vi "file list from temperatures file.vi"(11 "file path":path=path "/snowfall/Users/arcadi/Desktop/Ultrasound/Experiment/YBCO_4/Round1/Sweep12/June_2011/062511/221.16400K_300_3100_001_062511.dat") -> (0 "timestamp":dbl[](array[numeric]), 2 "sweep file name array":T1[](array[typedef]), 3 "temperatures":dbl[](array[numeric]))   [LabVIEW 2010]
uses:
  sweep file name.ctl
  <vilib>/regexp/Match Regular Expression.xnode
  <vilib>/Utility/file.llb/Read From Spreadsheet File (string).vi
panel:
  in  "dummy 2":T1={"temperature"=0.0, "temperature str"="", "file path"=path "/snowfall/Users/arcadi/Desktop/Ultrasound/Experiment/YBCO_4/Round1/Sweep12/June_2011/062511/221.16400K_300_3100_001_062511.dat", "last mod"=timestamp(0 s since 1904-01-01), "file name str"="", "mod time(min)"=0.0}
  in  "dummy":T1={"temperature"=0.0, "temperature str"="", "file path"=path "/snowfall/Users/arcadi/Desktop/Ultrasound/Experiment/YBCO_4/Round1/Sweep12/June_2011/062511/221.16400K_300_3100_001_062511.dat", "last mod"=timestamp(0 s since 1904-01-01), "file name str"="", "mod time(min)"=0.0}
  in  "sweep file name":T1={"temperature"=0.0, "temperature str"="", "file path"=path "/snowfall/Users/arcadi/Desktop/Ultrasound/Experiment/YBCO_4/Round1/Sweep12/June_2011/062511/221.16400K_300_3100_001_062511.dat", "last mod"=timestamp(0 s since 1904-01-01), "file name str"="", "mod time(min)"=0.0}
  in  "file path OK":bool=TRUE
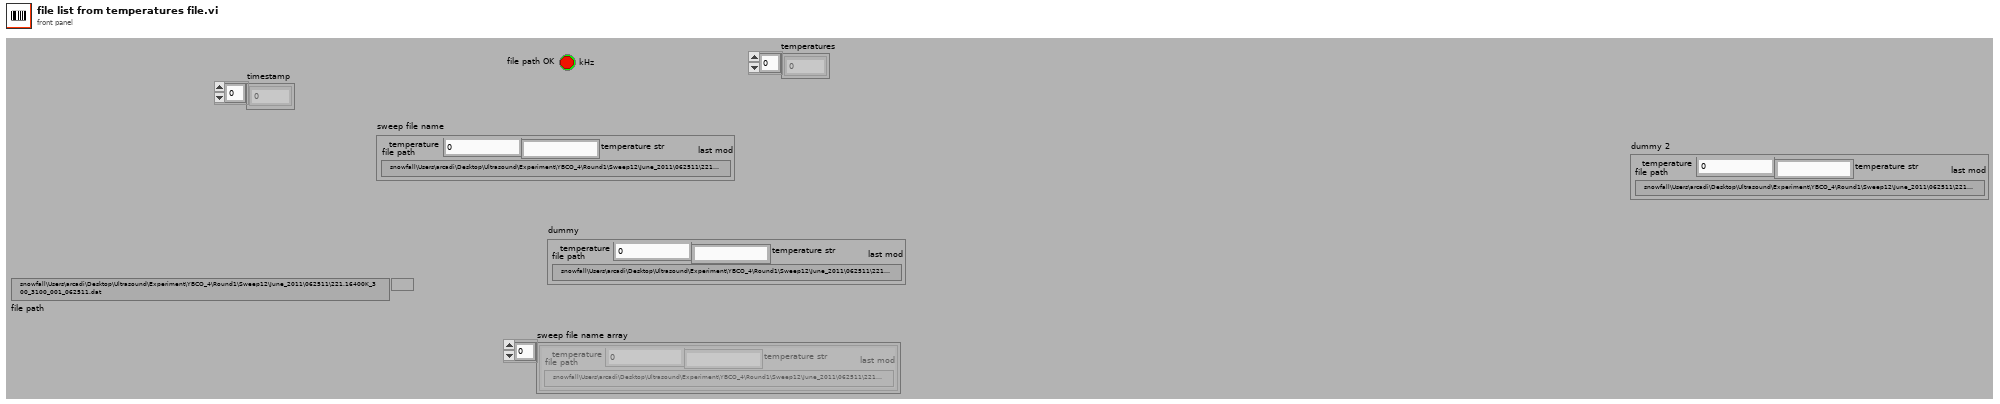
[diagram p1: front panel]
types:
  T1 = typedef "sweep file name.ctl" = cluster{"temperature":dbl, "temperature str":string, "file path":path, "last mod":timestamp, "file name str":string, "mod time(min)":dbl}
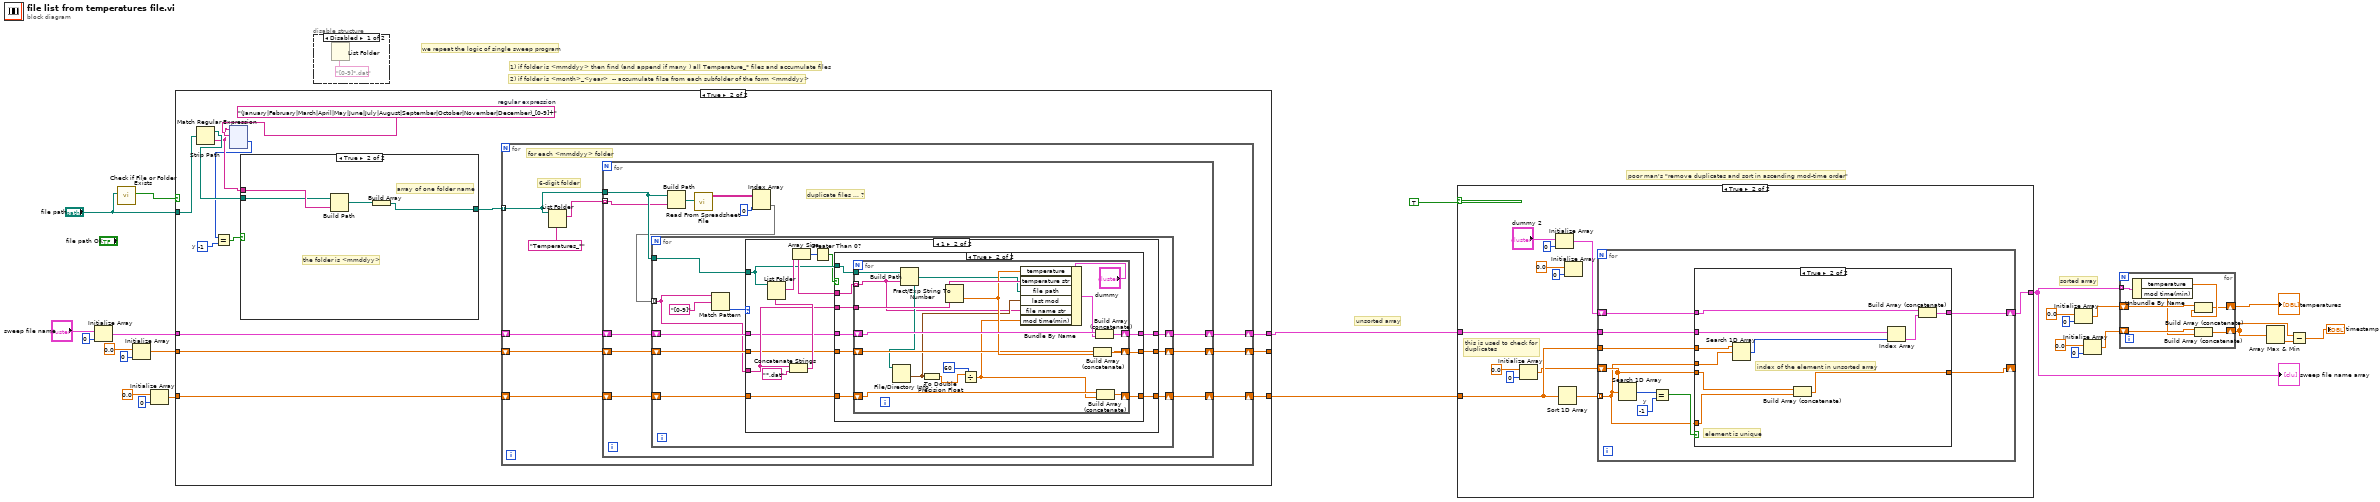
[diagram p0: block diagram]
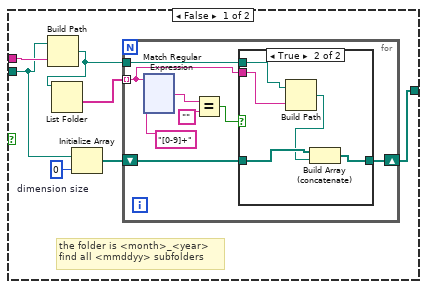
[diagram p6: hidden frame]
diagram:
  # "sorted array"
  # "unsorted array"
  # "poor man's \"remove duplicates and sort in ascending mod-time order\""
  # "1) if folder is <mmddyy> then find (and append if many ) all Temperature_* files and accumulate files"
  # "2) if folder is <month>_<year>  -- accumulate filse from each subfolder of the form <mmddyy>"
  # "we repeat the logic of single sweep program"
  n1 = Initialize Array("sweep file name", 0 ("dimension size")) -> (w19:T1[])
  n2 = call <vilib>:"Check if File or Folder Exists.vi"("path"="file path") -> ("file or folder exists?"=w24:bool)  [unwired: 8 in, 2 out]
  n3 = Initialize Array(0.0 ("dimension size"), 0 ("dimension size")) -> (w18:dbl[])
  n4 = Initialize Array(0.0 ("dimension size"), 0 ("dimension size")) -> (w15:dbl[])
  n5 = case shown="True" w24 {
    tunnel: "file path" -> [_ w38]
    tunnel: [w28 w40] -> w11
    tunnel: [w27 w39] -> _
    tunnel: w19 -> [w28 w42]
    tunnel: w18 -> [w27 w41]
    tunnel: w15 -> [w26 w36]
    tunnel: [w26 w35] -> w12
    frame False {
    }
    frame True {
      w30 = -1  # y
      w33 = "(January|February|March|April|May|June|July|August|September|October|November|December)_[0-9]+"  # regular expression
      n6 = Strip Path(path=w38) -> (stripped path=w34:path, name=w32:string)
      n7 = xnode "Match Regular Expression"("input string"=w32, "regular expression"=w33) -> ("offset past match"=w31:i32)  [unwired: 4 in, 4 out]
      n8 = Equal?(x=w31, y=w30) -> (x = y?=w29:bool)
      n9 = case shown="True" w29 {
        tunnel: w32 -> [w160 w289]
        tunnel: w34 -> [w158 w288]
        tunnel: [w154 w286] -> w37
        frame False {
          w157 = 0  # dimension size
          # "the folder is <month>_<year>\nfind all <mmddyy> subfolders"
          n10 = Build Path(base path=w158, name or relative path=w160) -> (appended path=w155:path)
          n11 = List Folder(path=w155) -> (folder names=w159:string[])  [unwired: 3 in, 3 out]
          n12 = Initialize Array(w158, w157) -> (w156:path[])
          n13 = for {
            tunnel: w159 -> [w161] mode=indexing
            shift-right: [w162] -> w154
            shift-left: w156 -> [w163]
            tunnel: w155 -> [w164]
            n14 = xnode "Match Regular Expression"("input string"=w161, "regular expression"="[0-9]+") -> ("after match"=w167:string)  [unwired: 4 in, 4 out]
            n15 = Equal?(x=w167, y="") -> (x = y?=w165:bool)
            n16 = case shown="True" w165 {
              tunnel: w164 -> [_ w285]
              tunnel: w161 -> [_ w284]
              tunnel: w163 -> [w280 w283]
              tunnel: [w280 w281] -> w162
              frame False {
              }
              frame True {
                n17 = Build Path(base path=w285, name or relative path=w284) -> (appended path=w282:path)
                n18 = Build Array (concatenate)(w283, w282) -> (w281:path[])
              }
            }
          }
        }
        frame True {
          # "the folder is <mmddyy>"
          # "array of one folder name"
          n19 = Build Path(base path=w288, name or relative path=w289) -> (appended path=w287:path)
          n20 = Build Array(w287) -> (w286:path[])
        }
      }
      n21 = for {
        tunnel: w37 -> [w295] mode=indexing
        shift-right: [w293] -> w40
        shift-left: w42 -> [w296]
        shift-right: [w294] -> w39
        shift-left: w41 -> [w292]
        shift-right: [w290] -> w35
        shift-left: w36 -> [w291]
        # "6-digit folder"
        # "for each <mmddyy> folder"
        n22 = List Folder(path=w295, pattern="Temperatures_*") -> (filenames=w297:string[])  [unwired: 2 in, 3 out]
        n23 = for {
          tunnel: w297 -> [w301] mode=indexing
          tunnel: w295 -> [w309]
          shift-right: [w303] -> w293
          shift-left: w296 -> [w310]
          shift-right: [w308] -> w294
          shift-left: w292 -> [w302]
          shift-right: [w299] -> w290
          shift-left: w291 -> [w300]
          # "duplicate files ... ?"
          n24 = Build Path(base path=w309, name or relative path=w301) -> (appended path=w307:path)
          n25 = call-poly <vilib>:"Read From Spreadsheet File.vi"("file path (dialog if empty)"=w307) -> ("all rows"=w306:string[][])  [unwired: 6 in, 4 out]
          n26 = Index Array(array=w306, index (col)=0 ("disabled index (col)")) -> (element=w304:string[])  [unwired: 1 in]
          n27 = for {
            tunnel: w304 -> [w315] mode=indexing
            tunnel: w309 -> [w320]
            shift-right: [w318] -> w303
            shift-left: w310 -> [w319]
            shift-right: [w316] -> w308
            shift-left: w302 -> [w317]
            shift-right: [w311] -> w299
            shift-left: w300 -> [w312]
            n28 = Match Pattern(string=w315, regular expression="[0-9]") -> (offset past match=w313:i32)  [unwired: 1 in, 3 out]
            n29 = case shown="1" w313 {
              tunnel: w320 -> [_ w333]
              tunnel: w315 -> [_ w332]
              tunnel: w319 -> [w322 w331]
              tunnel: [w322 w330] -> w318
              tunnel: w317 -> [w323 w329]
              tunnel: [w323 w328] -> w316
              tunnel: w312 -> [w321 w327]
              tunnel: [w321 w326] -> w311
              frame -1, Default {
              }
              frame 1 {
                n30 = Concatenate Strings(w332, "*.dat" ("string")) -> (w335:string)
                n31 = List Folder(path=w333, pattern=w335) -> (filenames=w334:string[])  [unwired: 2 in, 3 out]
                n32 = Array Size(array=w334) -> (size(s)=w325:i32)
                n33 = Greater Than 0?(x=w325) -> (x > 0?=w324:bool)
                n34 = case shown="True" w324 {
                  tunnel: w334 -> [_ w348]
                  tunnel: w333 -> [_ w347]
                  tunnel: w332 -> [_ w346]
                  tunnel: w331 -> [w339 w345]
                  tunnel: [w339 w342] -> w330
                  tunnel: w329 -> [w338 w344]
                  tunnel: [w338 w341] -> w328
                  tunnel: w327 -> [w337 w343]
                  tunnel: [w337 w340] -> w326
                  frame False {
                    # "duplicat tempearture folder"
                  }
                  frame True {
                    n35 = for {
                      tunnel: w348 -> [w352] mode=indexing
                      tunnel: w347 -> [w365]
                      tunnel: w346 -> [w363]
                      shift-right: [w355] -> w342
                      shift-left: w345 -> [w362]
                      shift-right: [w354] -> w341
                      shift-left: w344 -> [w359]
                      shift-right: [w353] -> w340
                      shift-left: w343 -> [w357]
                      n36 = Build Path(base path=w365, name or relative path=w352) -> (appended path=w358:path)
                      n37 = File/Directory Info(path=w358) -> (last mod=w356:timestamp)  [unwired: 1 in, 6 out]
                      n38 = To Double Precision Float(number=w356) -> (double precision float=w351:dbl)
                      n39 = Fract/Exp String To Number(string=w363) -> (number=w360:dbl)  [unwired: 3 in, 1 out]
                      n40 = Divide(x=w351, y=60) -> (x/y=w349:dbl)
                      n41 = Bundle By Name(cluster="dummy", "temperature"=w360, "temperature str"=w363, "file path"=w358, "last mod"=w356, "file name str"=w352, "mod time(min)"=w349) -> (w361:T1)
                      n42 = Build Array (concatenate)(w359, w360) -> (w354:dbl[])
                      n43 = Build Array (concatenate)(w362, w361) -> (w355:T1[])
                      n44 = Build Array (concatenate)(w357, w349) -> (w353:dbl[])
                    }
                  }
                }
              }
            }
          }
        }
      }
    }
  }
  n45 = disable-structure shown="Disabled" {
    frame Disabled {
      n46 = List Folder(pattern="[0-9]*.dat") -> ()  [unwired: 3 in, 4 out]
    }
    frame Enabled {
    }
  }
  n47 = case shown="True" TRUE {
    tunnel: w12 -> [_ w371]
    tunnel: w11 -> [w367 w378]
    tunnel: [w367 w377] -> w1
    frame False {
    }
    frame True {
      # "this is used to check for \nduplicates"
      n48 = Initialize Array(0.0 ("dimension size"), 0 ("dimension size")) -> (w368:dbl[])
      n49 = Initialize Array("dummy 2", 0 ("dimension size")) -> (w372:T1[])
      n50 = Sort 1D Array(array=w371) -> (sorted array=w379:dbl[])
      n51 = Initialize Array(0.0 ("dimension size"), 0 ("dimension size")) -> ()  [unwired: 1 out]
      n52 = for {
        shift-right: [w386] -> w377
        shift-left: w372 -> [w385]
        shift-right: [w384] -> _
        shift-left: w368 -> [w383]
        tunnel: w379 -> [w380] mode=indexing
        tunnel: w371 -> [w382]
        tunnel: w378 -> [w381]
        w388 = -1  # y
        n53 = Search 1D Array(1D array=w383, element=w380) -> (index of element=w389:i32)  [unwired: 1 in]
        n54 = Equal?(x=w389, y=w388) -> (x = y?=w387:bool)
        n55 = case shown="True" w387 {
          tunnel: [w391 w400] -> w386
          tunnel: w385 -> [w391 w401]
          tunnel: [w390 w392] -> w384
          tunnel: w383 -> [w390 w394]
          tunnel: w382 -> [_ w399]
          tunnel: w380 -> [_ w398]
          tunnel: w381 -> [_ w396]
          tunnel: w380 -> [_ w393]
          frame False {
            # "element is not unique"
          }
          frame True {
            # "index of the element in unsorted array"
            # "element is unique"
            n56 = Search 1D Array(1D array=w399, element=w398) -> (index of element=w397:i32)  [unwired: 1 in]
            n57 = Build Array (concatenate)(w394, w393) -> (w392:dbl[])
            n58 = Index Array(array=w396, index=w397) -> (element=w395:T1)
            n59 = Build Array (concatenate)(w401, w395) -> (w400:T1[])
          }
        }
      }
    }
  }
  "sweep file name array" <- w1
  n60 = Initialize Array(0.0 ("dimension size"), 0 ("dimension size")) -> (w8:dbl[])
  n61 = Initialize Array(0.0 ("dimension size"), 0 ("dimension size")) -> (w5:dbl[])
  n62 = for {
    tunnel: w1 -> [w408] mode=indexing
    shift-right: [w402] -> w4
    shift-left: w8 -> [w406]
    shift-right: [w403] -> w3
    shift-left: w5 -> [w405]
    n63 = Unbundle By Name(w408) -> ("temperature"=w407:dbl, "mod time(min)"=w404:dbl)
    n64 = Build Array (concatenate)(w405, w404) -> (w403:dbl[])
    n65 = Build Array (concatenate)(w406, w407) -> (w402:dbl[])
  }
  "temperatures" <- w4
  n66 = Array Max & Min(array=w3) -> (min value=w14:dbl)  [unwired: 3 out]
  n67 = Subtract(x=w3, y=w14) -> (x-y=→"timestamp":dbl[])
